vi "Report Cal Measured Power.vi"(0 "CART TCP Connection In":refnum<k5>, 5 "Commit?":bool, 7 "Measured Cal Power":dbl caption="Power", 11 "error in (no error)":errorcluster) -> (4 "CART TCP Connection Out":refnum<k5>, 8 "TCP Messages":string[](array[string]), 14 "Command Sent":string, 15 "error out":errorcluster)   [LabVIEW 2011]
uses:
  WLAN/UUT/QCA/NART Constants.vi
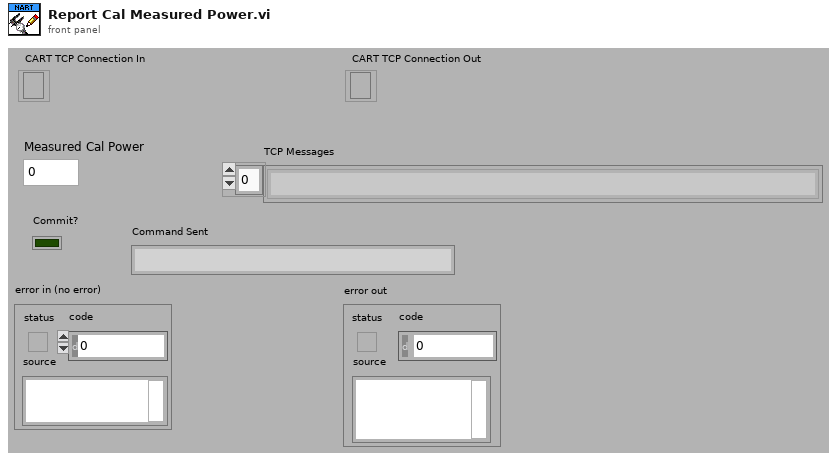
[diagram p1: front panel]
types:
  T1 = cluster{"Name":string, "Type":enum16{"decimal", "string", "float", "hex"}}[]
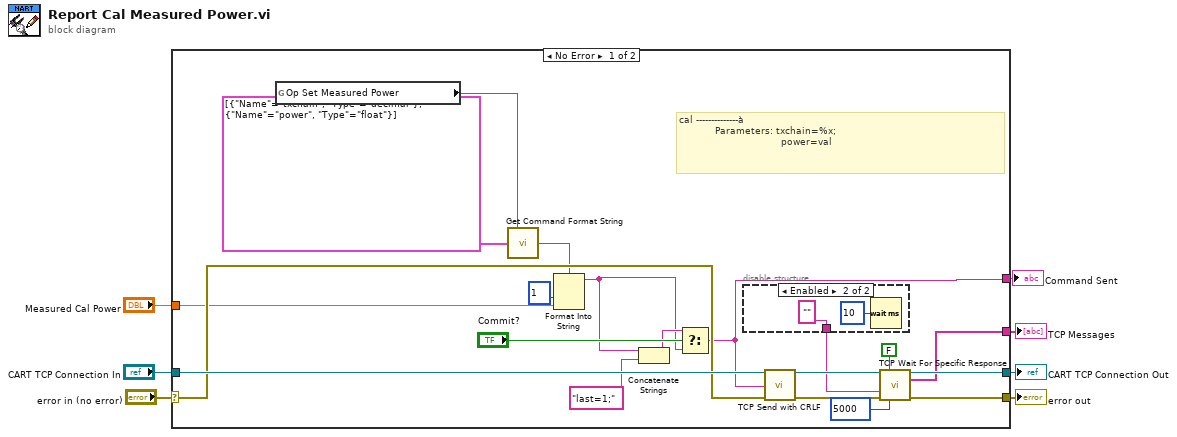
[diagram p0: block diagram]
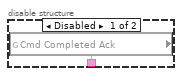
[diagram p2: hidden frame]
diagram:
  n1 = case shown="No Error" "error in (no error)" {
    selector: "error in (no error)" -> [w25 w32]
    tunnel: [w22 w32] -> w6
    tunnel: "CART TCP Connection In" -> [w27 w31]
    tunnel: [w23 w31] -> w4
    tunnel: [w19 _] -> w3
    tunnel: "Measured Cal Power" -> [w14 _]
    tunnel: [w10 _] -> w1
    frame No Error {
      # "cal --------------à\n            Parameters: txchain=%x;\n                                  power=val"
      n2 = global read "NART Constants.vi" "Op Set Measured Power"() -> (w17:string)
      n3 = call "Get Command Format String.vi"("Command"=w17, "Parameters"=T1 [{"Name"="txchain", "Type"=enum."decimal"}, {"Name"="power", "Type"=enum."float"}]) -> ("Command Format String"=w16:string)  [unwired: 13 in]
      n4 = Format Into String(format string=w16, u32 1 ("input 1"), w14) -> (resulting string=w8:string)  [unwired: 2 in, 1 out]
      n5 = Concatenate Strings(w8, "last=1;" ("string")) -> (w9:string)
      n6 = Select(t=w9, s="Commit?", f=w8) -> (s? t:f=w10:string)
      n7 = disable-structure shown="Enabled" {
        disable-tunnel: [w28 "" ("Expected Message Start (\"\":any)")] -> w13
        frame Disabled {
          n8 = global read "NART Constants.vi" "Cmd Completed Ack"() -> (w28:string)
        }
        frame Enabled {
          n9 = Wait (ms)(milliseconds to wait=u32 10) -> ()  [unwired: 1 out]
        }
      }
      n10 = call "TCP Send with CRLF.vi"("CART TCP Connection"=w27, "data in"=w10, "error IO"=w25) -> ("CART TCP Connection Out"=w24:refnum<k5>, "error out"=w21:errorcluster)  [unwired: 11 in]
      n11 = call "TCP Wait For Specific Response.vi"("TCP Connection In"=w24, "Next response (t)"=FALSE, "Expected Message Start (\"\":any)"=w13, "error in"=w21, "Timeout (250 ms)"=5000) -> ("TCP Connection Out"=w23:refnum<k5>, "TCP Messages"=w19:string[], "error out"=w22:errorcluster)  [unwired: 7 in, 1 out]
    }
    frame Error {
    }
  }
  "error out" <- w6
  "CART TCP Connection Out" <- w4
  "TCP Messages" <- w3
  "Command Sent" <- w1
